vi "CT400_testwrap.vi"() -> ()   [LabVIEW 2009]
uses:
  CT400_lib.lvlib
panel:
  out "Error Init":i32
  in  "LaserType":u32(ring) items=["LS_TunicsPlus", "LS_TunicsPurity", "LS_TunicsReference", "LS_TunicsT100s_HP", "LS_TunicsT100r", "LS_JdsuSws", "LS_Agilent", "NB_SOURCE"]
  out "CT400 option":string
  out "# Spectral Lines":i32
  out "Spectral lines":dbl[](array[numeric]) format="%#.4f"
  in  "Resolution [pm]":u32 max=128 step=1
  out "#Nb of available \ndetectors":i32
  out "# Nb of available\ninputs":i32
  out "# of acquired points":i32
  out "Vext out":dbl format="%.4g"
  out "# of resampled points":i32
  out "Pout-interpolated":dbl[](array[numeric]) format="%.2g"
  out "Detector-interpolated":dbl[](array[numeric]) format="%.2g"
  out "Wavelength re-sampled":dbl[](array[numeric]) format="%.3g"
  in  "Interpolated data":string
  in  "Re-sampled wavelength":string
  in  "Detector data":string
  in  "Wavelength data":string
  out "Pout":dbl[](array[numeric]) format="%.2g"
  out "Detector":dbl[](array[numeric]) format="%#.2g"
  out "Wavelength":dbl[](array[numeric]) format="%.4f"
  out "P4 [dBm]":dbl format="%.2g"
  out "P3 [dBm]":dbl format="%.2g"
  out "P2 [dBm]":dbl format="%.2g"
  out "P1 [dBm]":dbl format="%.2g"
  out "Pout [dBm]":dbl format="%.2g"
  out "Error/warning":string
  out "error out":errorcluster
  in  "Start Wavelength [nm]":dbl
  in  "Laser power output [mW]":dbl
  in  "Stop Wavelength [nm]":dbl
  in  "Speed [nm/s]":i32
  in  "GPIB Address":i32
  in  "Upper Wavelength [nm]":dbl
  in  "Lower Wavelength [nm]":dbl
  in  "error in (no error)":errorcluster
  # "CT400 Settings"
  # "Data files (relative path)"
  # "Laser Settings"
  # "Power on detectors"
  # "Re-sampled Measurements"
  # "Measurements"
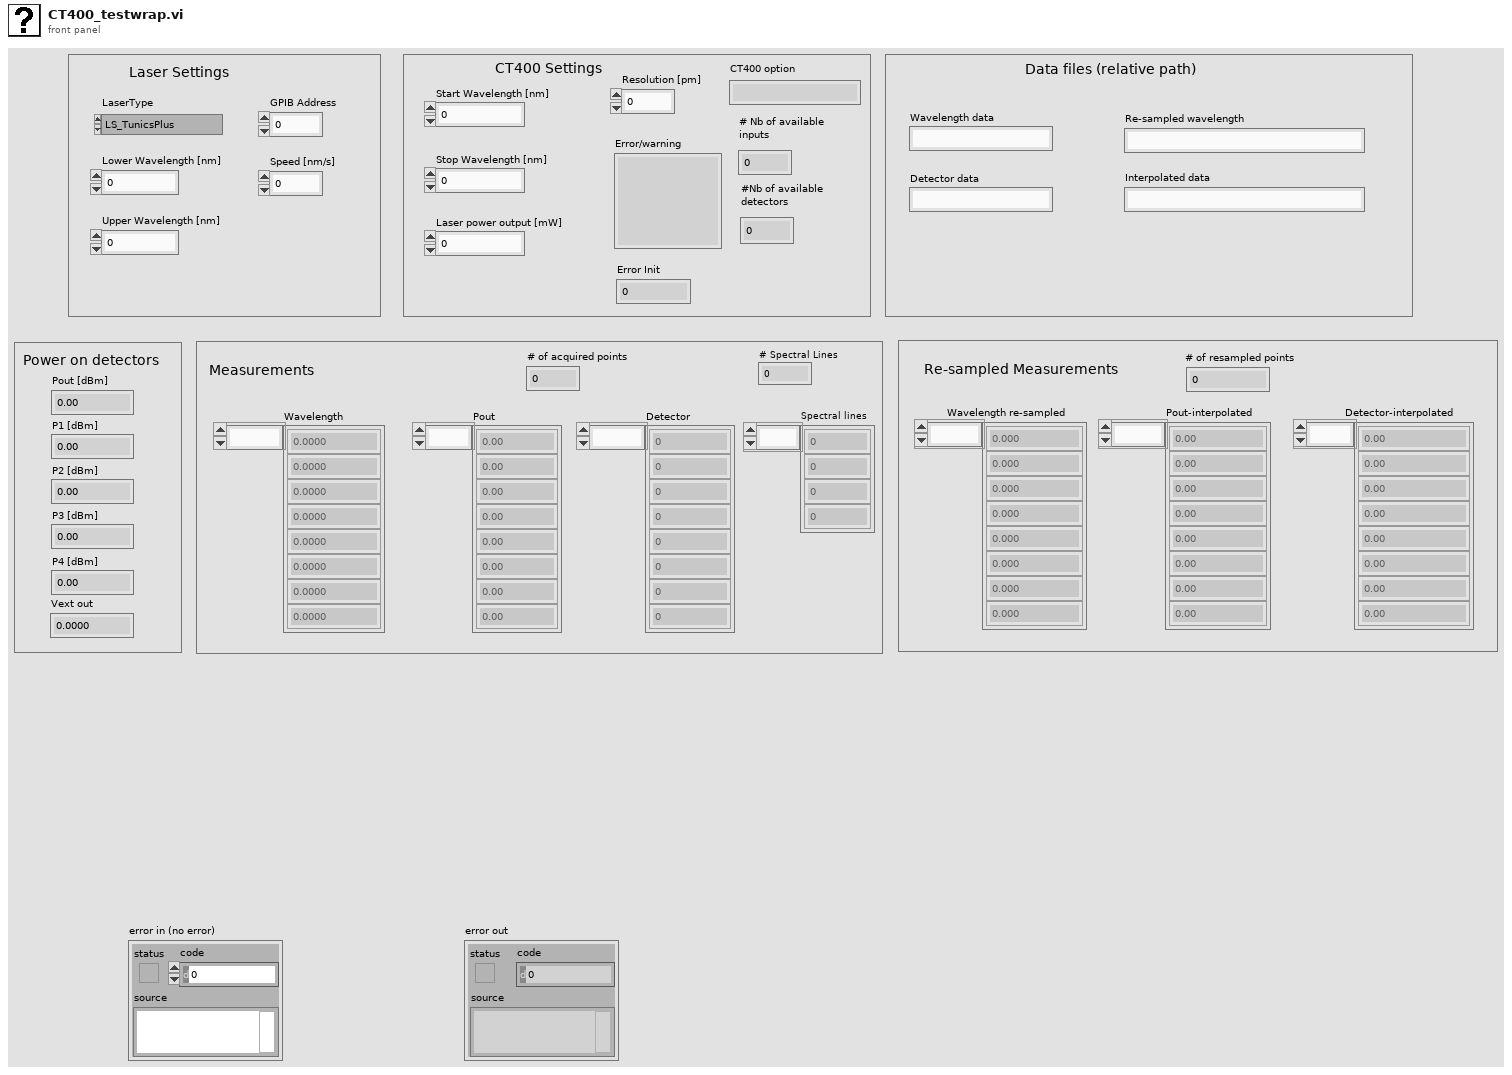
[diagram p1: front panel]
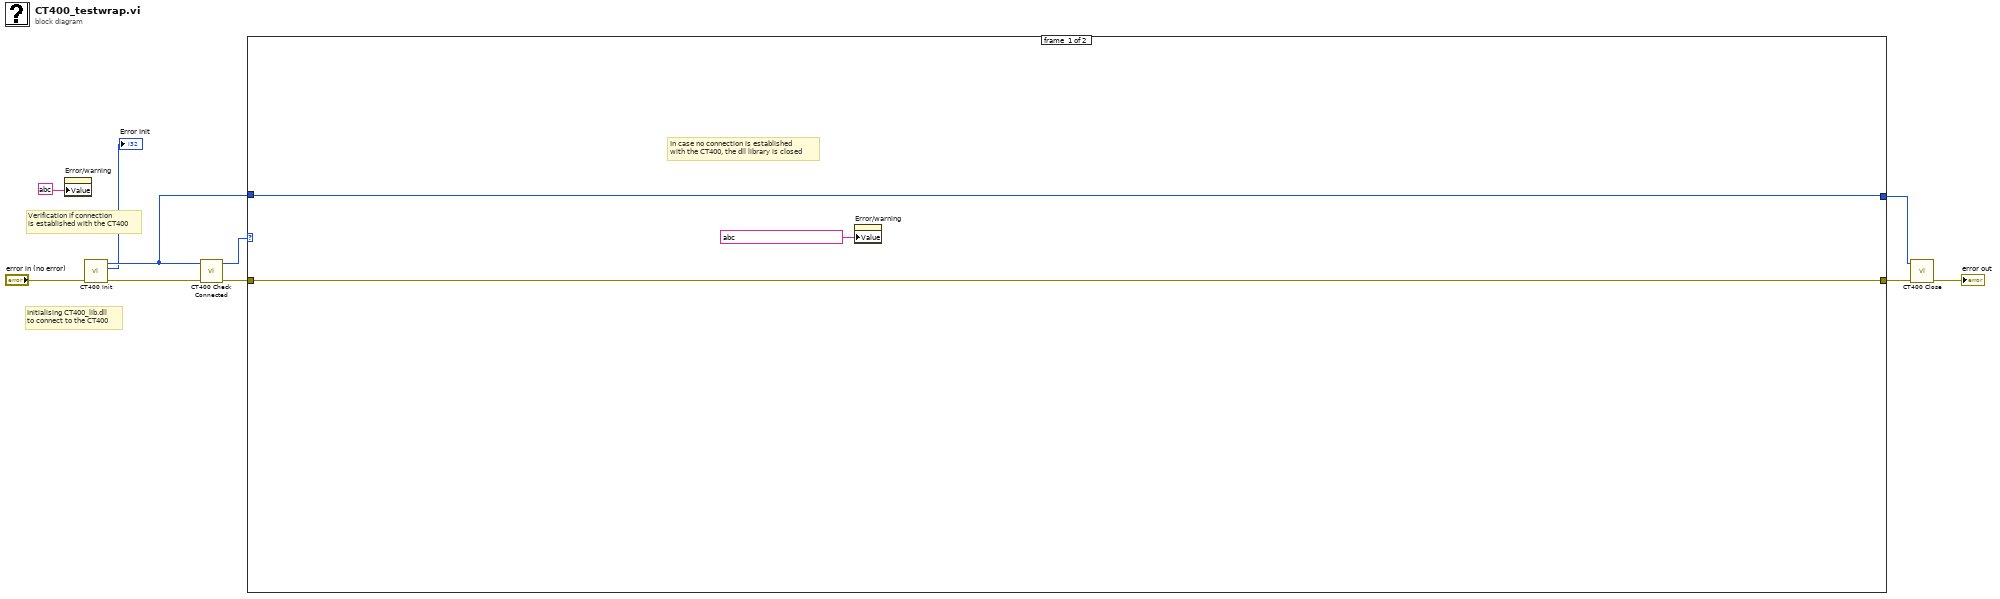
[diagram p0: block diagram]
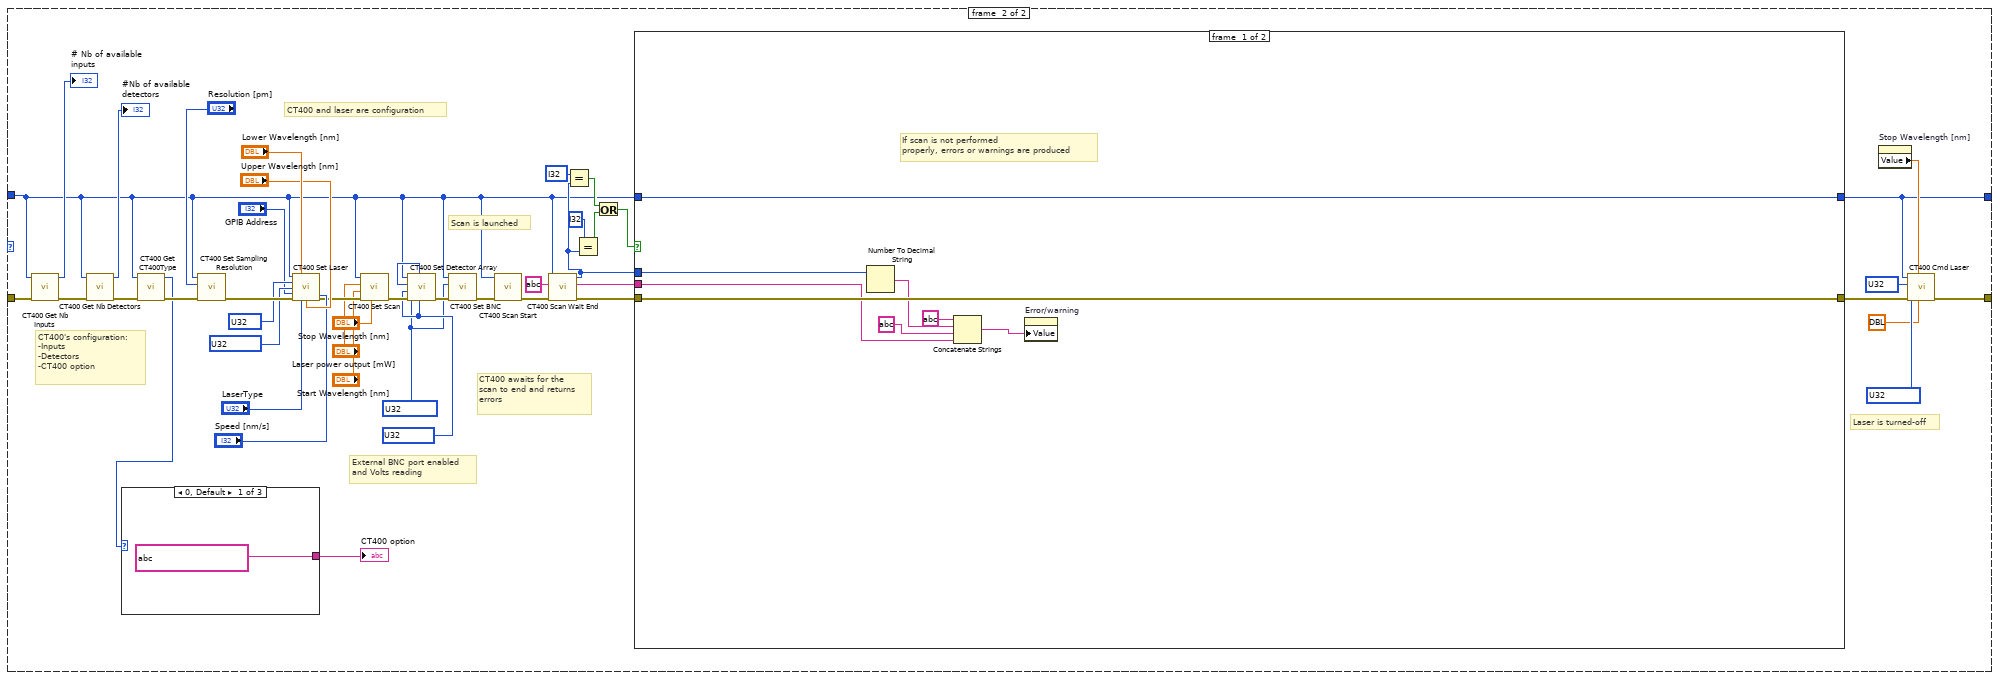
[diagram p2: hidden frame]
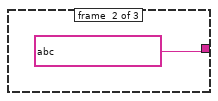
[diagram p3: hidden frame]
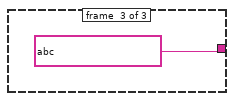
[diagram p4: hidden frame]
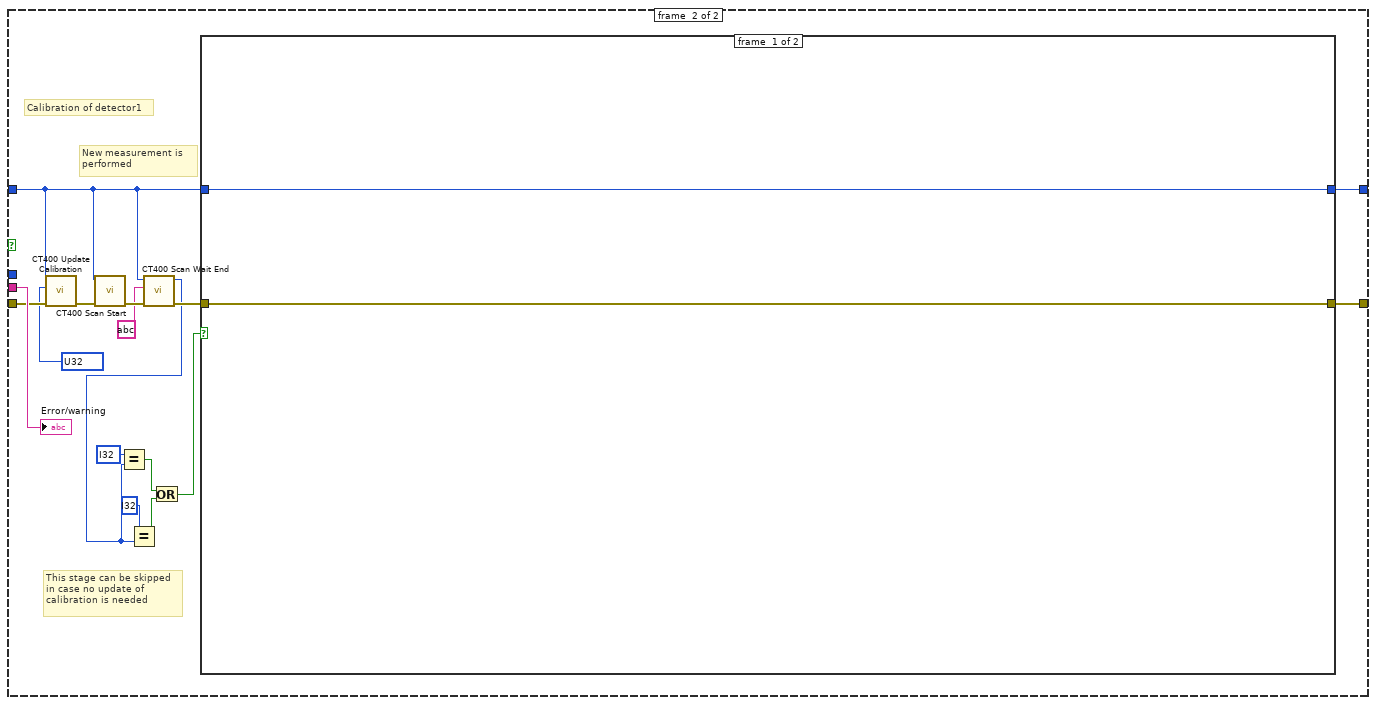
[diagram p5: hidden frame]
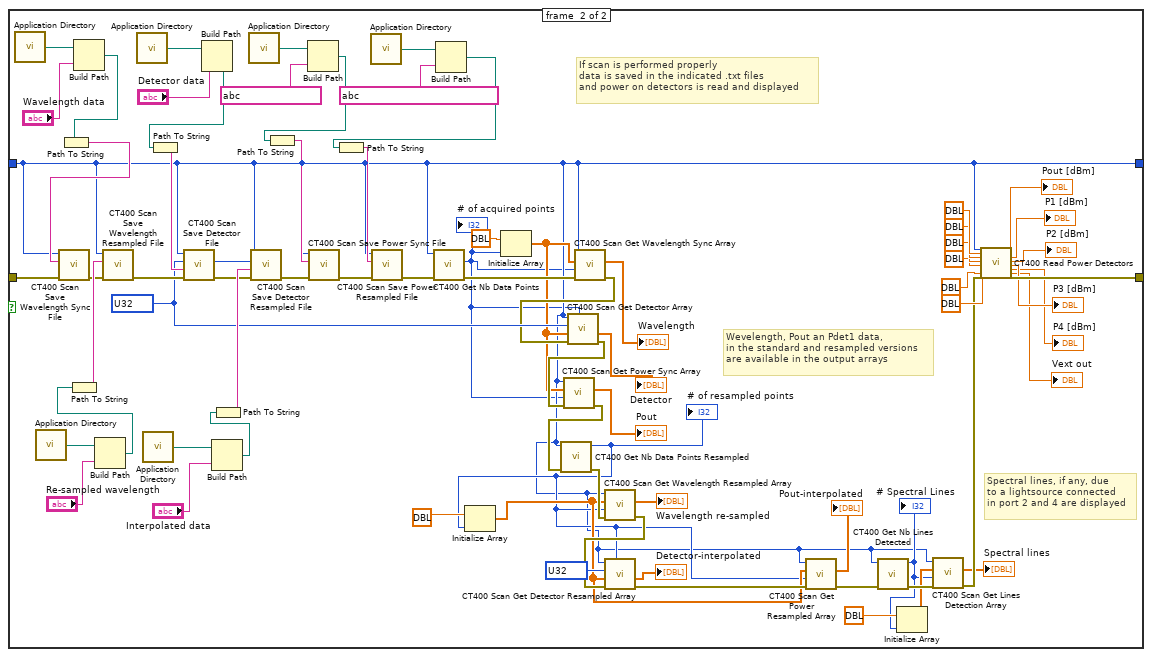
[diagram p6: hidden frame]
diagram:
  # "Verification if connection\nis established with the CT400"
  # "Initialising CT400_lib.dll\nto connect to the CT400"
  n1 = property on="Error/warning" class="Str"("Value"=string ?) -> ()  [unwired: 2 in, 2 out]
  n2 = call "CT400 Init.vi"("error in (no error)"="error in (no error)") -> ("error out"=w4:errorcluster, "iError out"=→"Error Init":i32, "function return"=w3:u64)  [unwired: 6 in]
  n3 = call "CT400 Check Connected.vi"("error in (no error)"=w4, "uiHandle"=w3) -> ("error out"=w8:errorcluster, "function return"=w9:i32)  [unwired: 8 in]
  n4 = case shown="1" w9 {
    tunnel: [w13 w42] -> w7
    tunnel: w8 -> [w13 w29]
    tunnel: w3 -> [w11 w15]
    tunnel: [w11 w17] -> w2
    frame #0 {
      # "In case no connection is established\nwith the CT400, the dll library is closed"
      n5 = property on="Error/warning" class="Str"("Value"=string ? ("Error/warning")) -> ()  [unwired: 2 in, 2 out]
    }
    frame #1 {
      w19 = u32 ? items=["DISABLE", "ENABLE"] ("eDect4")
      w16 = u32 ? items=["DISABLE", "ENABLE"] ("eDect4")
      w40 = u32 ? items=["LI_1", "LI_2", "LI_3", "LI_4"] ("eLaser")
      w41 = u32 ? items=["DISABLE", "ENABLE"] ("eEnable")
      w55 = u32 ? items=["DISABLE", "ENABLE"] ("eEnable")
      w56 = u32 ? items=["LI_1", "LI_2", "LI_3", "LI_4"] ("eLaser")
      # "CT400's configuration:\n-Inputs\n-Detectors\n-CT400 option"
      # "External BNC port enabled\nand Volts reading"
      # "Laser is turned-off"
      # "CT400 awaits for the\nscan to end and returns\nerrors"
      # "Scan is launched"
      # "CT400 and laser are configuration"
      n6 = call "CT400 Get Nb Inputs.vi"("error in (no error)"=w29, "uiHandle"=w15) -> ("error out"=w27:errorcluster, "function return"=→"# Nb of available\ninputs":i32)  [unwired: 8 in]
      n7 = call "CT400 Get Nb Detectors.vi"("error in (no error)"=w27, "uiHandle"=w15) -> ("error out"=w24:errorcluster, "function return"=→"#Nb of available \ndetectors":i32)  [unwired: 8 in]
      n8 = call "CT400 Get CT400Type.vi"("error in (no error)"=w24, "uiHandle"=w15) -> ("error out"=w23:errorcluster, "function return"=w22:i32)  [unwired: 8 in]
      n9 = case shown="0, Default" w22 {
        tunnel: [string ? ("CT400 option") string ? ("CT400 option") string ? ("CT400 option")] -> w21
        frame #0 {
        }
        frame #1 {
        }
        frame #2 {
        }
      }
      "CT400 option" <- w21
      n10 = call "CT400 Set Sampling Resolution.vi"("error in (no error)"=w23, "uiResolution"="Resolution [pm]", "uiHandle"=w15) -> ("error out"=w57:errorcluster)  [unwired: 7 in, 1 out]
      n11 = call "CT400 Set Laser.vi"("uiHandle"=w15, "eLaserType"="LaserType", "dMaxWavelength"="Upper Wavelength [nm]", "eLaser"=w56, "eEnable"=w55, "iGPIBAdress"="GPIB Address", "error in (no error)"=w57, "dMinWavelength"="Lower Wavelength [nm]", "Speed"="Speed [nm/s]") -> ("error out"=w50:errorcluster)  [unwired: 5 in, 1 out]
      n12 = call "CT400 Set Scan.vi"("dMaxWavelength"="Stop Wavelength [nm]", "error in (no error)"=w50, "dMinWavelength"="Start Wavelength [nm]", "dLaserPower"="Laser power output [mW]", "uiHandle"=w15) -> ("error out"=w30:errorcluster)  [unwired: 5 in, 1 out]
      n13 = call "CT400 Set Detector Array.vi"("eExt"=w19, "eDect4"=w16, "error in (no error)"=w30, "eDect3"=w19, "eDect2"=w16, "uiHandle"=w15) -> ("error out"=w18:errorcluster)  [unwired: 4 in, 1 out]
      n14 = call "CT400 Set BNC.vi"("error in (no error)"=w18, "eEnable"=w16, "uiHandle"=w15) -> ("error out"=w14:errorcluster)  [unwired: 7 in, 1 out]
      n15 = call "CT400 Scan Start.vi"("error in (no error)"=w14, "uiHandle"=w15) -> ("error out"=w31:errorcluster)  [unwired: 8 in, 1 out]
      n16 = call "CT400 Scan Wait End.vi"("error in (no error)"=w31, "tcError"=string ?, "uiHandle"=w15) -> ("error out"=w45:errorcluster, "tcError out"=w44:string, "function return"=w36:i32)  [unwired: 6 in]
      n17 = Equal?(x=i32 ?, y=w36) -> (x = y?=w33:bool)
      n18 = Equal?(x=i32 ?, y=w36) -> (x = y?=w34:bool)
      n19 = Or(x=w33, y=w34) -> (x .or. y?=w32:bool)
      n20 = case shown="True" w32 {
        tunnel: [w68 w83] -> w43
        tunnel: w45 -> [w68 w82]
        tunnel: w44 -> [w65 w84]
        tunnel: w36 -> [w67 _]
        tunnel: w15 -> [w61 w70]
        tunnel: [w61 w69] -> w17
        frame #0 {
          # "If scan is not performed \nproperly, errors or warnings are produced"
          n21 = Number To Decimal String(number=w67) -> (decimal integer string=w66:string)  [unwired: 1 in]
          n22 = Concatenate Strings(string ? ("string"), w66, string ? ("string"), w65) -> (w64:string)
          n23 = property on="Error/warning" class="Str"("Value"=w64) -> ()  [unwired: 2 in, 2 out]
        }
        frame #1 {
          w81 = u32 ? items=["DE_1", "DE_2", "DE_3", "DE_4", "DE_5"] ("eDetector")
          # "New measurement is \nperformed"
          # "This stage can be skipped\nin case no update of \ncalibration is needed"
          # "Calibration of detector1"
          n24 = call "CT400 Update Calibration.vi"("error in (no error)"=w82, "eDetector"=w81, "uiHandle"=w70) -> ("error out"=w80:errorcluster)  [unwired: 7 in, 1 out]
          n25 = call "CT400 Scan Start.vi"("error in (no error)"=w80, "uiHandle"=w70) -> ("error out"=w79:errorcluster)  [unwired: 8 in, 1 out]
          n26 = call "CT400 Scan Wait End.vi"("error in (no error)"=w79, "tcError"=string ?, "uiHandle"=w70) -> ("error out"=w78:errorcluster, "function return"=w72:i32)  [unwired: 6 in, 1 out]
          n27 = Equal?(x=i32 ?, y=w72) -> (x = y?=w76:bool)
          n28 = Equal?(x=i32 ?, y=w72) -> (x = y?=w75:bool)
          n29 = Or(x=w76, y=w75) -> (x .or. y?=w71:bool)
          n30 = case shown="True" w71 {
            tunnel: [w86 w157] -> w83
            tunnel: w78 -> [w86 w89]
            tunnel: w70 -> [w85 w88]
            tunnel: [w85 w88] -> w69
            frame #0 {
            }
            frame #1 {
              w126 = u32 ? items=["DE_1", "DE_2", "DE_3", "DE_4", "DE_5"] ("eDetector")
              w129 = u32 ? items=["DE_1", "DE_2", "DE_3", "DE_4"] ("Detector")
              # "Spectral lines, if any, due\nto a lightsource connected\nin port 2 and 4 are displayed"
              # "Wevelength, Pout an Pdet1 data,\nin the standard and resampled versions\nare available in the output arrays"
              # "If scan is performed properly\ndata is saved in the indicated .txt files\nand power on detectors is read and displayed"
              n31 = call <vilib>:"Application Directory.vi"() -> ("Application Directory"=w90:path)
              n32 = call <vilib>:"Application Directory.vi"() -> ("Application Directory"=w140:path)
              n33 = Build Path(base path=w90, name or relative path="Wavelength data") -> (appended path=w144:path)
              n34 = Path To String(path=w144) -> (string=w159:string)
              n35 = call "CT400 Scan Save Wavelength Sync File.vi"("error in (no error)"=w89, "pcPath"=w159, "uiHandle"=w88) -> ("error out"=w136:errorcluster)  [unwired: 6 in, 2 out]
              n36 = Build Path(base path=w140, name or relative path="Re-sampled wavelength") -> (appended path=w138:path)
              n37 = Path To String(path=w138) -> (string=w137:string)
              n38 = call "CT400 Scan Save Wavelength Resampled File.vi"("error in (no error)"=w136, "pcPath"=w137, "uiHandle"=w88) -> ("error out"=w135:errorcluster)  [unwired: 6 in, 2 out]
              n39 = call <vilib>:"Application Directory.vi"() -> ("Application Directory"=w143:path)
              n40 = call <vilib>:"Application Directory.vi"() -> ("Application Directory"=w134:path)
              n41 = Build Path(base path=w143, name or relative path="Detector data") -> (appended path=w141:path)
              n42 = Path To String(path=w141) -> (string=w158:string)
              n43 = call "CT400 Scan Save Detector File.vi"("error in (no error)"=w135, "pcPath"=w158, "eDetector"=w129, "uiHandle"=w88) -> ("error out"=w130:errorcluster)  [unwired: 5 in, 2 out]
              n44 = Build Path(base path=w134, name or relative path="Interpolated data") -> (appended path=w132:path)
              n45 = Path To String(path=w132) -> (string=w131:string)
              n46 = call <vilib>:"Application Directory.vi"() -> ("Application Directory"=w112:path)
              n47 = call "CT400 Scan Save Detector Resampled File.vi"("error in (no error)"=w130, "pcPath"=w131, "eDetector"=w129, "uiHandle"=w88) -> ("error out"=w118:errorcluster)  [unwired: 5 in, 2 out]
              n48 = Build Path(base path=w112, name or relative path=string ?) -> (appended path=w113:path)
              n49 = Path To String(path=w113) -> (string=w109:string)
              n50 = call "CT400 Scan Save Power Sync File.vi"("error in (no error)"=w118, "pcPath"=w109, "uiHandle"=w88) -> ("error out"=w117:errorcluster)  [unwired: 6 in, 2 out]
              n51 = call <vilib>:"Application Directory.vi"() -> ("Application Directory"=w114:path)
              n52 = Build Path(base path=w114, name or relative path=string ?) -> (appended path=w115:path)
              n53 = Path To String(path=w115) -> (string=w108:string)
              n54 = call "CT400 Scan Save Power Resampled File.vi"("error in (no error)"=w117, "pcPath"=w108, "uiHandle"=w88) -> ("error out"=w116:errorcluster)  [unwired: 6 in, 2 out]
              n55 = call "CT400 Get Nb Data Points.vi"("error in (no error)"=w116, "uiHandle"=w88) -> ("error out"=w120:errorcluster, "iDataPoints out"=w87:i32)  [unwired: 6 in, 2 out]
              "# of acquired points" <- w87
              n56 = Initialize Array(dbl ? ("element"), w87) -> (w104:dbl[])
              n57 = call "CT400 Scan Get Wavelength Sync Array.vi"("error in (no error)"=w120, "iArraySize"=w87, "dArray"=w104, "uiHandle"=w88) -> ("error out"=w119:errorcluster, "dArray out"=→"Wavelength":dbl[])  [unwired: 5 in, 1 out]
              n58 = call "CT400 Scan Get Detector Array.vi"("iArraySize"=w87, "error in (no error)"=w119, "dArray"=w104, "eDetector"=w129, "uiHandle"=w88) -> ("error out"=w146:errorcluster, "dArray out"=→"Detector":dbl[])  [unwired: 4 in, 1 out]
              n59 = call "CT400 Scan Get Power Sync Array.vi"("error in (no error)"=w146, "iArraySize"=w87, "dArray"=w104, "uiHandle"=w88) -> ("error out"=w103:errorcluster, "dArray out"=→"Pout":dbl[])  [unwired: 5 in, 1 out]
              n60 = call "CT400 Get Nb Data Points Resampled.vi"("error in (no error)"=w103, "uiHandle"=w88) -> ("error out"=w102:errorcluster, "function return"=w99:i32)  [unwired: 8 in]
              "# of resampled points" <- w99
              n61 = Initialize Array(dbl ? ("element"), w99) -> (w101:dbl[])
              n62 = call "CT400 Scan Get Wavelength Resampled Array.vi"("error in (no error)"=w102, "iArraySize"=w99, "dArray"=w101, "uiHandle"=w88) -> ("error out"=w128:errorcluster, "dArray out"=→"Wavelength re-sampled":dbl[])  [unwired: 5 in, 1 out]
              n63 = call "CT400 Scan Get Detector Resampled Array.vi"("iArraySize"=w99, "error in (no error)"=w128, "dArray"=w101, "eDetector"=w126, "uiHandle"=w88) -> ("error out"=w127:errorcluster, "dArray out"=→"Detector-interpolated":dbl[])  [unwired: 4 in, 1 out]
              n64 = call "CT400 Scan Get Power Resampled Array.vi"("error in (no error)"=w127, "iArraySize"=w99, "dArray"=w101, "uiHandle"=w88) -> ("error out"=w98:errorcluster, "dArray out"=→"Pout-interpolated":dbl[])  [unwired: 5 in, 1 out]
              n65 = call "CT400 Get Nb Lines Detected.vi"("error in (no error)"=w98, "uiHandle"=w88) -> ("error out"=w97:errorcluster, "function return"=w94:i32)  [unwired: 8 in]
              "# Spectral Lines" <- w94
              n66 = Initialize Array(dbl ? ("element"), w94) -> (w95:dbl[])
              n67 = call "CT400 Scan Get Lines Detection Array.vi"("error in (no error)"=w97, "iArraySize"=w94, "dArray"=w95, "uiHandle"=w88) -> ("error out"=w93:errorcluster, "dArray out"=→"Spectral lines":dbl[])  [unwired: 5 in, 1 out]
              n68 = call "CT400 Read Power Detectors.vi"("uiHandle"=w88, "Pout"=dbl ?, "P1"=dbl ?, "P2"=dbl ?, "P3"=dbl ?, "P4"=dbl ?, "Vext"=dbl ?, "error in (no error)"=w93) -> ("Pout out"=→"Pout [dBm]":dbl, "P1 out"=→"P1 [dBm]":dbl, "P2 out"=→"P2 [dBm]":dbl, "P3 out"=→"P3 [dBm]":dbl, "P4 out"=→"P4 [dBm]":dbl, "Vext out"=→"Vext out":dbl, "error out"=w157:errorcluster)  [unwired: 12 in, 1 out]
            }
          }
          "Error/warning" <- w84
        }
      }
      n69 = property on="Stop Wavelength [nm]" class="DigNum (strict)"() -> ("Value"=w38:dbl)  [unwired: 2 in, 2 out]
      n70 = call "CT400 Cmd Laser.vi"("dPower"=dbl ?, "dWavelength"=w38, "error in (no error)"=w43, "eEnable"=w41, "eLaser"=w40, "uiHandle"=w17) -> ("error out"=w42:errorcluster)  [unwired: 4 in, 1 out]
    }
  }
  n71 = call "CT400 Close.vi"("error in (no error)"=w7, "uiHandle"=w2) -> ("error out"=→"error out":errorcluster)  [unwired: 8 in, 1 out]
